vi "camera_synchrone_acquisition.vi"() -> ()   [LabVIEW 2018]
uses:
  <userlib>/WaveKit.lib/Controls/Image information.ctl
  <userlib>/WaveKit.lib/Controls/Image general information.ctl
  <userlib>/WaveKit.lib/Controls/Image acquisition information.ctl
  <userlib>/WaveKit.lib/Controls/Point2D.ctl
  <userlib>/WaveKit.lib/Controls/Data alignment enum.ctl
  <userlib>/WaveKit.lib/Classes/Camera/Camera.lvclass
  <userlib>/WaveKit.lib/Classes/CameraSet/CameraSet.lvclass
  <userlib>/WaveKit.lib/Classes/Image/Image.lvclass
panel:
  out "Acquisition information":T1={"Image general information"={"Camera serial number"="", "Smearing removed"=FALSE, "Background image removed"=FALSE, "Time Stamp"=timestamp(0 s since 1904-01-01), "Comment"="", "Camera_MAX_Level"=0}, "Acquisition information"={"Exposure duration (us)"=0, "Exposure duration specified (us)"=0, "Gain"=0.0, "Number of summed images"=0, "Trigger type"=""}, "Number of pixels"={"X"=0, "Y"=0}, "Number of bits"=enum."16"}
  in  "Init":bool
  in  "Reset error":bool
  in  "acquisition_mode":enum16{"last_image", "new_image"}(ring)
  out "exposure_duration_us (get)":u32
  in  "exposure_duration_us (set)":u32=1000 min=1
  out "Current error":errorcluster
  out "nb_image (get)":u32=10
  in  "nb_image (set)":u32=1 min=1
  in  "Show camera signal":bool
  in  "Exit":bool
  in  "Stop Acq":bool
  in  "Start Acq":bool
  out "Image Camera":u32[][](graph)
  in  "Configuration file path":path
  # "Acquisition Parameters"
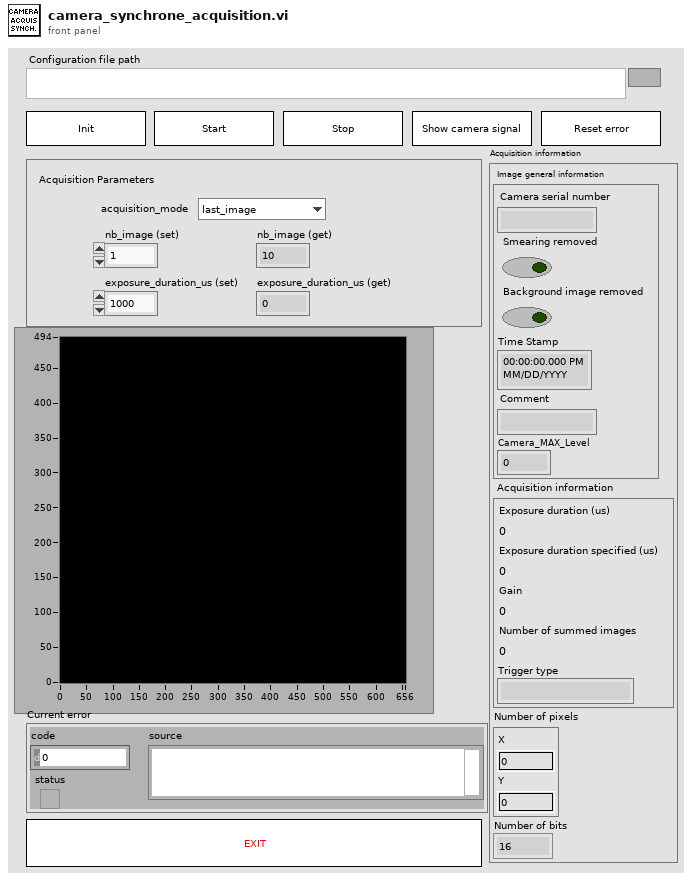
[diagram p1: front panel]
types:
  T1 = typedef "Image information.ctl" = cluster{"Image general information":T2, "Acquisition information":T3, "Number of pixels":T4, "Number of bits":T5}
  T2 = typedef "Image general information.ctl" = cluster{"Camera serial number":string, "Smearing removed":bool, "Background image removed":bool, "Time Stamp":timestamp, "Comment":string, "Camera_MAX_Level":i32}
  T3 = typedef "Image acquisition information.ctl" = cluster{"Exposure duration (us)":i32, "Exposure duration specified (us)":i32, "Gain":sgl, "Number of summed images":i32, "Trigger type":string}
  T4 = typedef "Point2D.ctl" = cluster{"X":u32, "Y":u32}
  T5 = typedef "Data alignment enum.ctl" = enum16{"8", "16", "32"}
  T6 = typedef "CameraSpecifications.ctl" = cluster{"Grabber name":string, "Camera name":string, "Camera sn":string, "Pixels_um":T7, "Maximum level":u32, "Data alignment":T5, "Is signed":bool, "Acquisition start":T4, "Acquisition length":T4, "MaxFrameRate_Hz":sgl, "Chip type":enum16{"Progressive scan", "Frame transfert"}}
  T7 = typedef "General dimensions definition.ctl" = cluster{"Size":T4, "Step":T8}
  T8 = typedef "Point2Df.ctl" = cluster{"X":sgl, "Y":sgl}
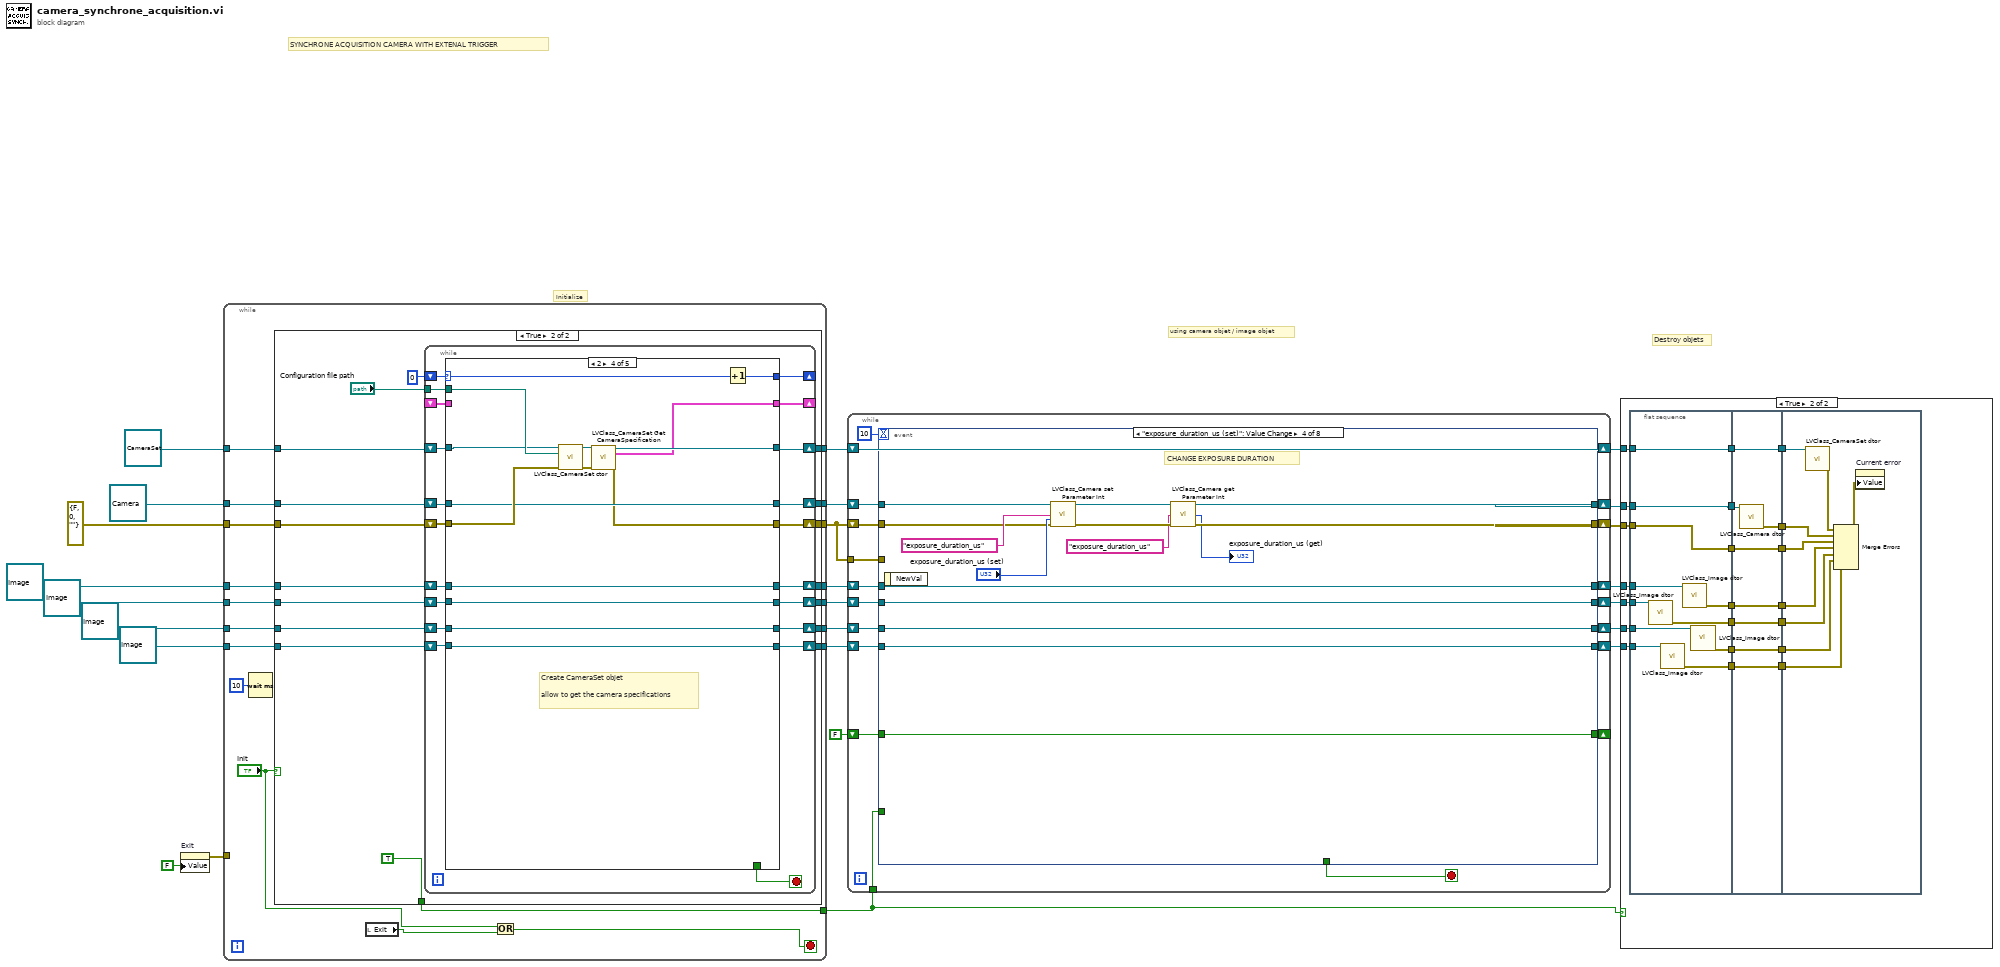
[diagram p0: block diagram]
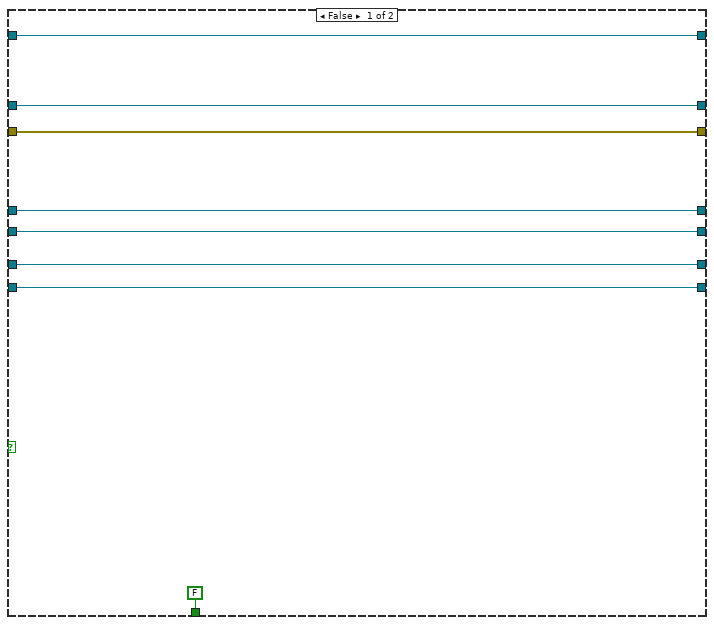
[diagram p3: hidden frame]
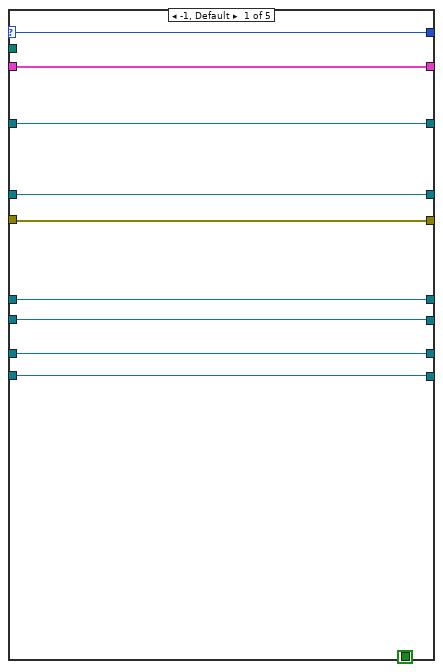
[diagram p4: hidden frame]
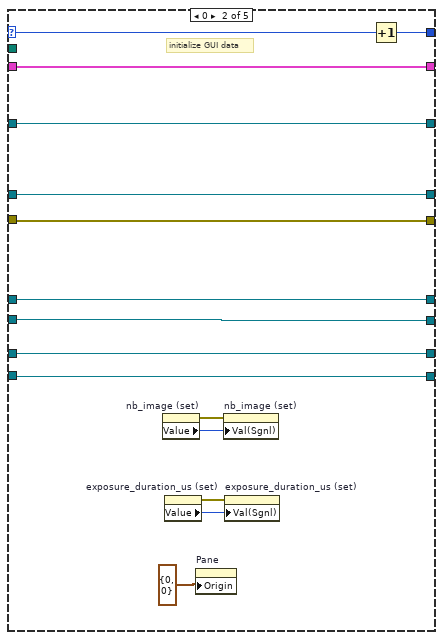
[diagram p5: hidden frame]
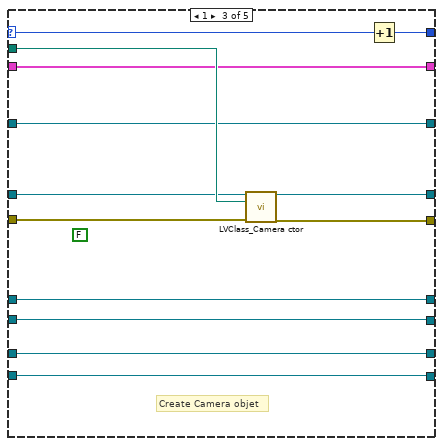
[diagram p6: hidden frame]
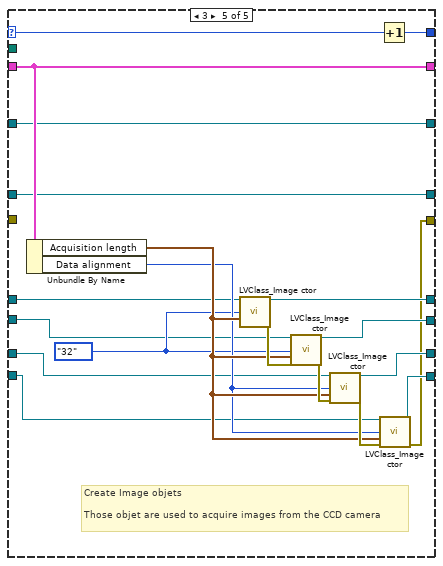
[diagram p7: hidden frame]
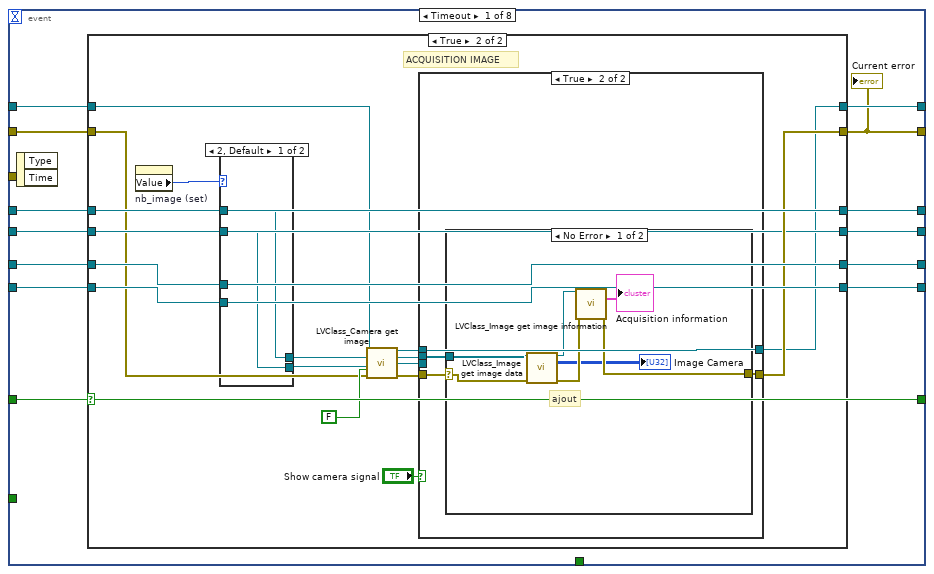
[diagram p8: hidden frame]
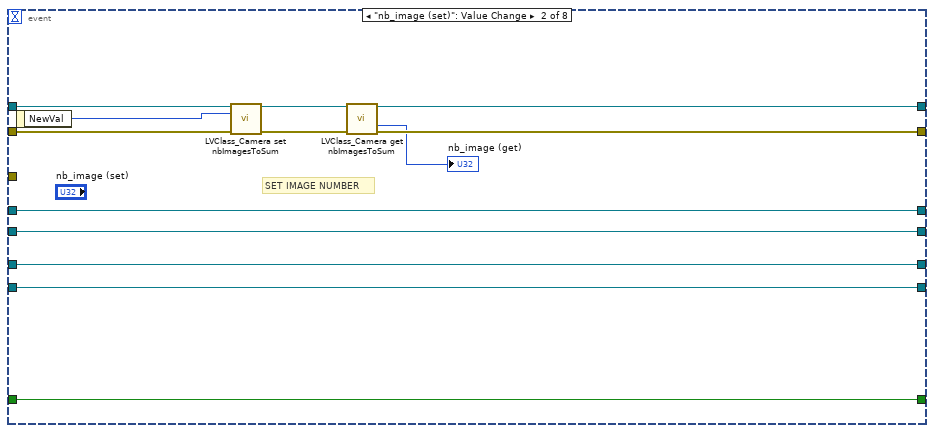
[diagram p13: hidden frame]
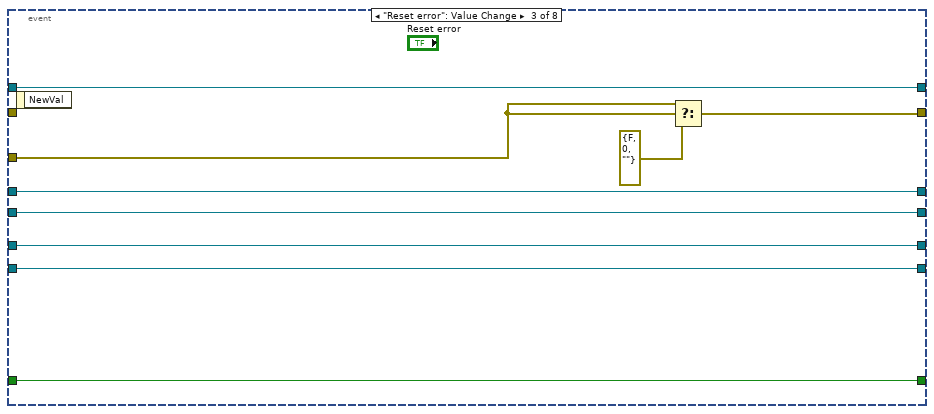
[diagram p14: hidden frame]
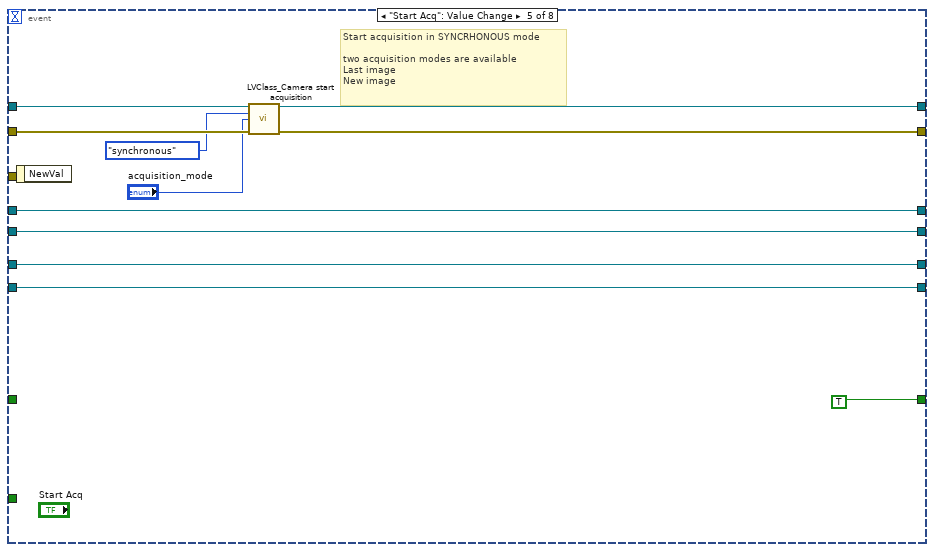
[diagram p15: hidden frame]
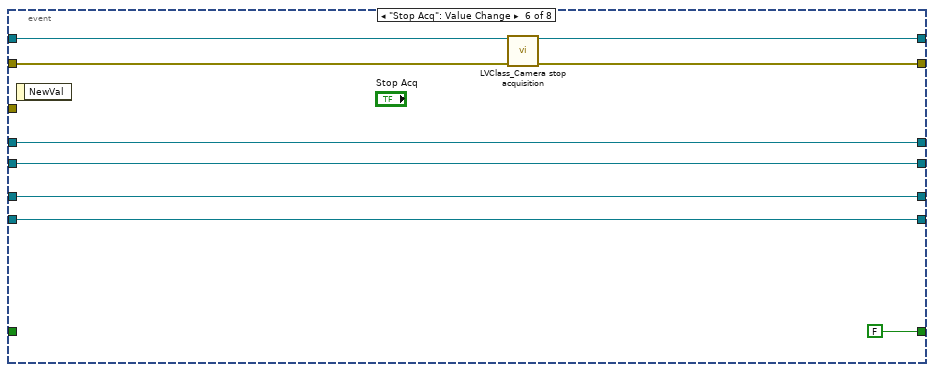
[diagram p16: hidden frame]
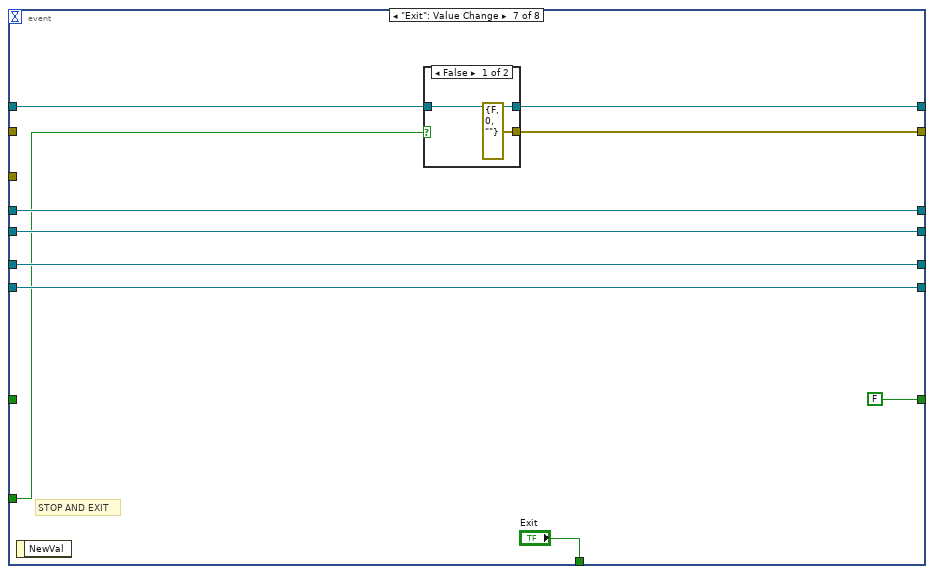
[diagram p17: hidden frame]
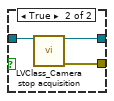
[diagram p18: hidden frame]
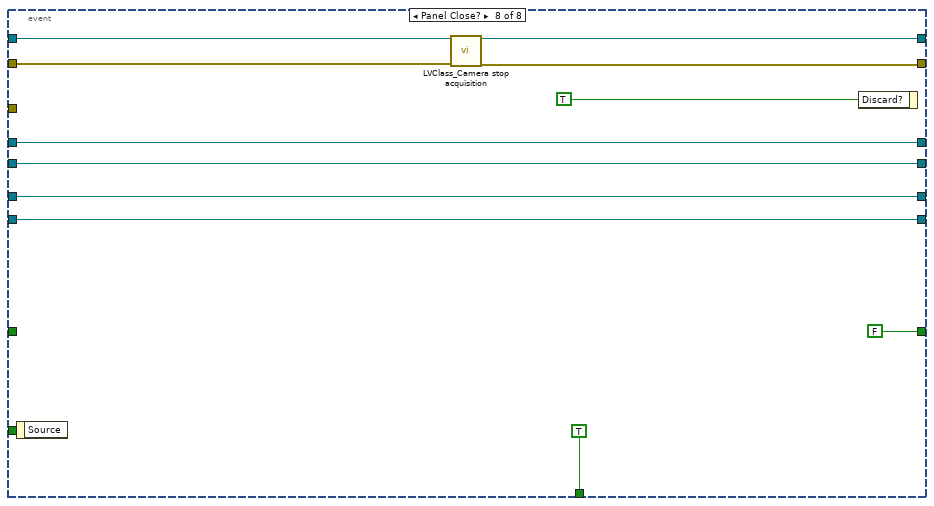
[diagram p19: hidden frame]
diagram:
  # "Destroy objets"
  # "using camera objet / image objet"
  # "Initialize"
  # "SYNCHRONE ACQUISITION CAMERA WITH EXTENAL TRIGGER"
  n1 = property on="Exit" class="Bool (strict)"("Value"=FALSE ("Exit")) -> (error out=w1:errorcluster)  [unwired: 2 in, 1 out]
  n2 = while {
    tunnel: [w44] -> w17
    tunnel: [w43] -> w16
    tunnel: [w42] -> w15
    tunnel: [w41] -> w14
    tunnel: [w40] -> w13
    tunnel: [w39] -> w12
    tunnel: refnum<class "Camera.lvclass"> refnum ("Camera.lvclass") -> [w38]
    tunnel: refnum<class "CameraSet.lvclass"> refnum ("CameraSet.lvclass") -> [w37]
    tunnel: refnum<class "Image.lvclass"> refnum ("Image in") -> [w36]
    tunnel: refnum<class "Image.lvclass"> refnum ("Image in") -> [w35]
    tunnel: refnum<class "Image.lvclass"> refnum ("Image in") -> [w34]
    tunnel: refnum<class "Image.lvclass"> refnum ("Image in") -> [w33]
    tunnel: errorcluster {"status"=FALSE, "code"=0, "source"=""} ("error out") -> [w32]
    tunnel: [w31] -> w4
    tunnel: [w27] -> w3
    tunnel: w1 -> [_]
    stop <- w28 stop-if-true
    n3 = Wait (ms)(milliseconds to wait=u32 10) -> ()  [unwired: 1 out]
    n4 = case shown="True" "Init" {
      tunnel: [w50 w69] -> w44
      tunnel: [w51 w68] -> w43
      tunnel: [w48 w66] -> w42
      tunnel: [w47 w65] -> w41
      tunnel: [w46 w64] -> w40
      tunnel: [w45 w63] -> w39
      tunnel: w38 -> [w50 w62]
      tunnel: w37 -> [w51 w60]
      tunnel: w36 -> [w48 w59]
      tunnel: w35 -> [w47 w58]
      tunnel: w34 -> [w46 w57]
      tunnel: w33 -> [w45 w56]
      tunnel: w32 -> [w49 w55]
      tunnel: [w49 w54] -> w31
      tunnel: [FALSE TRUE] -> w27
      frame False {
      }
      frame True {
        n5 = while {
          tunnel: "Configuration file path" -> [w87]
          shift-right: [w89] -> w69
          shift-left: w62 -> [w81]
          shift-right: [w71] -> _
          shift-left: 0 -> [w70]
          shift-right: [w88] -> w68
          shift-left: w60 -> [w80]
          shift-right: [w79] -> _
          shift-left: _ -> [w77]
          shift-right: [w86] -> w66
          shift-left: w59 -> [w78]
          shift-right: [w85] -> w65
          shift-left: w58 -> [w76]
          shift-right: [w84] -> w64
          shift-left: w57 -> [w74]
          shift-right: [w83] -> w63
          shift-left: w56 -> [w75]
          shift-right: [w82] -> w54
          shift-left: w55 -> [w72]
          stop <- w73 stop-if-true
          n6 = case shown="2" w70 {
            tunnel: [w99 w101 w127 w135 w149] -> w89
            tunnel: w87 -> [_ _ w126 w139 _]
            tunnel: [w98 w105 w124 w140 w150] -> w88
            tunnel: [w91 w106 w118 w130 w156] -> w86
            tunnel: [w92 w107 w119 w131 w155] -> w85
            tunnel: [w93 w108 w120 w132 w154] -> w84
            tunnel: [w94 w109 w121 w133 w153] -> w83
            tunnel: [w95 w100 w123 w134 w152] -> w82
            selector: w70 -> [w90 w103 w116 w129 w144]
            tunnel: w81 -> [w99 w101 w125 w135 w149]
            tunnel: w80 -> [w98 w105 w124 w138 w150]
            tunnel: [w96 w102 w122 w137 w151] -> w79
            tunnel: w78 -> [w91 w106 w118 w130 w148]
            tunnel: w77 -> [w96 w102 w122 _ w151]
            tunnel: w76 -> [w92 w107 w119 w131 w147]
            tunnel: w75 -> [w94 w109 w121 w133 w146]
            tunnel: w74 -> [w93 w108 w120 w132 w145]
            tunnel: [TRUE _ _ _ _] -> w73
            tunnel: w72 -> [w95 w100 w115 w136 _]
            tunnel: [w90 w104 w117 w128 w143] -> w71
            frame -1, Default {
            }
            frame 0 {
              # "initialize GUI data"
              n7 = property on="nb_image (set)" class="DigNum (strict)"() -> (error out=w114:errorcluster, "Value"=w113:u32)  [unwired: 2 in, 1 out]
              n8 = property on="exposure_duration_us (set)" class="DigNum (strict)"() -> (error out=w110:errorcluster, "Value"=w112:u32)  [unwired: 2 in, 1 out]
              n9 = property on="Pane" class="Pane"("Origin"=cluster{"Horizontal":i16, "Vertical":i16} {"Horizontal"=0, "Vertical"=0} ("Front Panel Window:Origin")) -> ()  [unwired: 2 in, 2 out]
              n10 = property on="nb_image (set)" class="DigNum (strict)"(error in=w114, "Val(Sgnl)"=w113) -> ()  [unwired: 1 in, 2 out]
              n11 = property on="exposure_duration_us (set)" class="DigNum (strict)"(error in=w110, "Val(Sgnl)"=w112) -> ()  [unwired: 1 in, 2 out]
              n12 = Increment(x=w103) -> (x+1=w104:i32)
            }
            frame 1 {
              (unwired) FALSE ("Acq required")
              # "Create Camera objet"
              n13 = call <userlib>:"LVClass_Camera ctor.vi"("Camera"=w125, "Configuration file path"=w126, "error in (no error)"=w115) -> ("Camera (new)"=w127:refnum<class "Camera.lvclass">, "error out"=w123:errorcluster)  [unwired: 11 in]
              n14 = Increment(x=w116) -> (x+1=w117:i32)
            }
            frame 2 {
              # "Create CameraSet objet\n\nallow to get the camera specifications"
              n15 = call <userlib>:"LVClass_CameraSet ctor.vi"("CameraSet.lvclass"=w138, "Configuration file path"=w139, "error in (no error)"=w136) -> ("CameraSet.lvclass"=w142:refnum<class "CameraSet.lvclass">, "error out"=w141:errorcluster)  [unwired: 11 in]
              n16 = call <userlib>:"LVClass_CameraSet Get CameraSpecification.vi"("CameraSet.lvclass"=w142, "error in (no error)"=w141) -> ("CameraSet.lvclass"=w140:refnum<class "CameraSet.lvclass">, "Camera Config"=w137:T6, "error out"=w134:errorcluster)  [unwired: 11 in]
              n17 = Increment(x=w129) -> (x+1=w128:i32)
            }
            frame 3 {
              w157 = Data_alignment_enum."32" ("Data alignment")
              # "Create Image objets\n\nThose objet are used to acquire images from the CCD camera"
              n18 = Unbundle By Name(w151) -> ("Acquisition length"=w159:T4, "Data alignment"=w158:T5)
              n19 = call <userlib>:"LVClass_Image ctor.vi"("Image in"=w148, "Data alignment"=w157, "Size"=w159) -> ("Image out"=w156:refnum<class "Image.lvclass">, "error out"=w160:errorcluster)  [unwired: 11 in]
              n20 = call <userlib>:"LVClass_Image ctor.vi"("Image in"=w147, "Data alignment"=w157, "Size"=w159, "error in (no error)"=w160) -> ("Image out"=w155:refnum<class "Image.lvclass">, "error out"=w161:errorcluster)  [unwired: 10 in]
              n21 = call <userlib>:"LVClass_Image ctor.vi"("Image in"=w145, "Data alignment"=w158, "Size"=w159, "error in (no error)"=w161) -> ("Image out"=w154:refnum<class "Image.lvclass">, "error out"=w162:errorcluster)  [unwired: 10 in]
              n22 = Increment(x=w144) -> (x+1=w143:i32)
              n23 = call <userlib>:"LVClass_Image ctor.vi"("Image in"=w146, "Data alignment"=w158, "Size"=w159, "error in (no error)"=w162) -> ("Image out"=w153:refnum<class "Image.lvclass">, "error out"=w152:errorcluster)  [unwired: 10 in]
            }
          }
        }
      }
    }
    n24 = local read "Exit"() -> (w29:bool)
    n25 = Or(x="Init", y=w29) -> (x .or. y?=w28:bool)
  }
  n26 = while {
    shift-right: [w178] -> w25
    shift-left: w4 -> [w180]
    shift-right: [w176] -> w24
    shift-left: w17 -> [w177]
    shift-right: [w170] -> w23
    shift-left: w15 -> [w175]
    shift-right: [w169] -> w22
    shift-left: w14 -> [w174]
    shift-right: [w168] -> w21
    shift-left: w13 -> [w173]
    shift-right: [w167] -> w20
    shift-left: w12 -> [w172]
    shift-right: [w166] -> _
    shift-left: FALSE -> [w171]
    shift-right: [w165] -> w19
    shift-left: w16 -> [w165]
    tunnel: w4 -> [w164]
    tunnel: w3 -> [w163]
    stop <- w179 stop-if-true
    n27 = event shown="[3] \"exposure_duration_us (set)\": Value Change" {
      selector: _ -> [_ _ _ _ _ _ _ _]
      dyn-events: _ -> [_ _ _ _ _ _ _ _]
      timeout: 10 -> [_ _ _ _ _ _ _ _]
      tunnel: w180 -> [w186 w247 _ w270 w282 w284 _ w309]
      tunnel: [_ _ _ _ _ _ "Exit" TRUE ("Exit")] -> w179
      tunnel: [w182 w245 w250 w265 w280 w290 w300 w314] -> w178
      tunnel: w177 -> [w191 w246 w252 w269 w283 w291 w301 w316]
      tunnel: [w190 w244 w252 w266 w281 w292 w299 w315] -> w176
      tunnel: w175 -> [w194 w237 w254 w259 w276 w286 w295 w310]
      tunnel: w174 -> [w193 w238 w255 w260 w275 w287 w296 w311]
      tunnel: w173 -> [w192 w239 w256 w261 w274 w288 w297 w312]
      tunnel: w172 -> [w187 w240 w257 w262 w273 w289 w298 w313]
      tunnel: w171 -> [w183 w236 w253 w258 _ _ _ _]
      tunnel: [w189 w237 w254 w259 w276 w286 w295 w310] -> w170
      tunnel: [w188 w238 w255 w260 w275 w287 w296 w311] -> w169
      tunnel: [w185 w239 w256 w261 w274 w288 w297 w312] -> w168
      tunnel: [w184 w240 w257 w262 w273 w289 w298 w313] -> w167
      tunnel: [w183 w236 w253 w258 TRUE FALSE FALSE FALSE] -> w166
      tunnel: w164 -> [_ _ w249 _ _ _ _ _]
      tunnel: w163 -> [_ _ _ _ _ _ w293 _]
      event Timeout {
        n28 = event-data() -> ()  [unwired: 1 in, 2 out]
        n29 = case shown="True" w183 {
          tunnel: [w195 w207] -> w182
          tunnel: w194 -> [w200 w213]
          tunnel: [w200 w213] -> w189
          tunnel: [w196 w204] -> w188
          tunnel: w192 -> [w199 w212]
          tunnel: w187 -> [w198 w211]
          tunnel: [w199 w212] -> w185
          tunnel: [w198 w211] -> w184
          tunnel: w193 -> [w196 w204]
          tunnel: w191 -> [w197 w203]
          tunnel: [w197 w202] -> w190
          tunnel: w186 -> [w195 w201]
          frame False {
          }
          frame True {
            # "ACQUISITION IMAGE"
            n30 = property on="nb_image (set)" class="DigNum (strict)"() -> ("Value"=w214:u32)  [unwired: 2 in, 2 out]
            n31 = case shown="2, Default" w214 {
              tunnel: [w219 w221] -> w215
              tunnel: w204 -> [w218 _]
              tunnel: w213 -> [w219 _]
              tunnel: [w218 w220] -> w210
              tunnel: w212 -> [_ w221]
              tunnel: w211 -> [_ w220]
              frame 2, Default {
              }
              frame 1 {
              }
            }
            n32 = call <userlib>:"LVClass_Camera get image.vi"("Camera in"=w203, "Image"=w215, "Image RAW"=w210, "remove_background"=FALSE, "error in (no error)"=w201) -> ("Camera out"=w217:refnum<class "Camera.lvclass">, "Image (dup)"=w208:refnum<class "Image.lvclass">, "Image (dup) RAW"=w209:refnum<class "Image.lvclass">, "error out"=w205:errorcluster)  [unwired: 7 in]
            n33 = case shown="True" "Show camera signal" {
              tunnel: w217 -> [w223 w224]
              tunnel: w208 -> [_ w225]
              tunnel: w205 -> [w222 w227]
              tunnel: [w223 w224] -> w202
              tunnel: [w222 w226] -> w207
              tunnel: w209 -> [_ _]
              frame False {
              }
              frame True {
                n34 = case shown="No Error" w227 {
                  selector: w227 -> [w234 w235]
                  tunnel: [w231 w235] -> w226
                  tunnel: w225 -> [w230 _]
                  frame No Error {
                    # "ajout"
                    n35 = call <userlib>:"LVClass_Image get image data.vi"("Image in"=w230, "error in (no error)"=w234) -> ("Image out"=w233:refnum<class "Image.lvclass">, "Image data out"=→"Image Camera":u32[][], "error out"=w232:errorcluster)  [unwired: 11 in]
                    n36 = call <userlib>:"LVClass_Image get image information.vi"("Image in"=w233, "error in (no error)"=w232) -> ("Acquisition information"=→"Acquisition information":T1, "error out"=w231:errorcluster)  [unwired: 11 in, 1 out]
                  }
                  frame Error {
                  }
                }
              }
            }
          }
        }
        "Current error" <- w182
      }
      event "nb_image (set)": Value Change {
        # "SET IMAGE NUMBER"
        n37 = event-data() -> ("NewVal"=w248:u32)  [unwired: 1 in]
        n38 = call <userlib>:"LVClass_Camera set nbImagesToSum.vi"("Camera in"=w246, "nb_image"=w248, "error in (no error)"=w247) -> ("Camera out"=w243:refnum<class "Camera.lvclass">, "error out"=w242:errorcluster)  [unwired: 11 in]
        n39 = call <userlib>:"LVClass_Camera get nbImagesToSum.vi"("Camera in"=w243, "error in (no error)"=w242) -> ("Camera out"=w244:refnum<class "Camera.lvclass">, "nb_image"=→"nb_image (get)":u32, "error out"=w245:errorcluster)  [unwired: 11 in]
      }
      event "Reset error": Value Change {
        n40 = event-data() -> ()  [unwired: 1 in, 1 out]
        n41 = Select(t=w249, s=w249, f=errorcluster {"status"=FALSE, "code"=0, "source"=""} ("error out")) -> (s? t:f=w250:errorcluster)
      }
      event "exposure_duration_us (set)": Value Change {
        # "CHANGE EXPOSURE DURATION"
        n42 = event-data() -> ()  [unwired: 1 in, 1 out]
        n43 = call <userlib>:"LVClass_Camera set Parameter Int.vi"("Camera in"=w269, "parameter_name"="exposure_duration_us", "value"="exposure_duration_us (set)", "error in (no error)"=w270) -> ("Camera out"=w268:refnum<class "Camera.lvclass">, "error out"=w267:errorcluster)  [unwired: 10 in]
        n44 = call <userlib>:"LVClass_Camera get Parameter Int.vi"("Camera in"=w268, "parameter_name"="exposure_duration_us", "error in (no error)"=w267) -> ("Camera out"=w266:refnum<class "Camera.lvclass">, "value"=→"exposure_duration_us (get)":i32, "error out"=w265:errorcluster)  [unwired: 10 in]
      }
      event "Start Acq": Value Change {
        # "Start acquisition in SYNCRHONOUS mode\n\ntwo acquisition modes are available\nLast image\nNew image"
        n45 = event-data() -> ()  [unwired: 1 in, 1 out]
        n46 = call <userlib>:"LVClass_Camera start acquisition.vi"("Camera in"=w283, "synchronisation_mode"=enum16{"synchronous", "asynchronous"}."synchronous", "acquisition_mode"="acquisition_mode", "error in (no error)"=w282) -> ("Camera out"=w281:refnum<class "Camera.lvclass">, "error out"=w280:errorcluster)  [unwired: 10 in]
      }
      event "Stop Acq": Value Change {
        n47 = event-data() -> ()  [unwired: 1 in, 1 out]
        n48 = call <userlib>:"LVClass_Camera stop acquisition.vi"("Camera in"=w291, "error in (no error)"=w284) -> ("Camera out"=w292:refnum<class "Camera.lvclass">, "error out"=w290:errorcluster)  [unwired: 12 in]
      }
      event "Exit": Value Change {
        # "STOP AND EXIT"
        n49 = event-data() -> ()  [unwired: 1 in, 1 out]
        n50 = case shown="False" w293 {
          tunnel: w301 -> [w304 w307]
          tunnel: [errorcluster {"status"=FALSE, "code"=0, "source"=""} ("error out") w306] -> w300
          tunnel: [w304 w305] -> w299
          frame False {
          }
          frame True {
            n51 = call <userlib>:"LVClass_Camera stop acquisition.vi"("Camera in"=w307) -> ("Camera out"=w305:refnum<class "Camera.lvclass">, "error out"=w306:errorcluster)  [unwired: 13 in]
          }
        }
      }
      event Panel Close? {
        n52 = event-data() -> ()  [unwired: 1 in, 1 out]
        n53 = call <userlib>:"LVClass_Camera stop acquisition.vi"("Camera in"=w316, "error in (no error)"=w309) -> ("Camera out"=w315:refnum<class "Camera.lvclass">, "error out"=w314:errorcluster)  [unwired: 12 in]
        n54 = event-data("Discard?"=TRUE) -> ()  [unwired: 1 in, 1 out]
      }
    }
  }
  n55 = case shown="True" w3 {
    tunnel: w25 -> [_ w325]
    tunnel: w24 -> [_ w324]
    tunnel: w23 -> [_ w323]
    tunnel: w22 -> [_ w322]
    tunnel: w21 -> [_ w321]
    tunnel: w20 -> [_ w320]
    tunnel: w19 -> [_ w319]
    frame False {
    }
    frame True {
      n56 = flat-sequence {
        tunnel: w324 -> [w350]
        tunnel: w325 -> [w348]
        tunnel: [w350] -> w339
        tunnel: w319 -> [w349]
        tunnel: [w349] -> w338
        tunnel: [w348] -> w337
        tunnel: w323 -> [w347]
        tunnel: w322 -> [w346]
        tunnel: w321 -> [w345]
        tunnel: w320 -> [w344]
        tunnel: [w343] -> w336
        tunnel: [w342] -> w335
        tunnel: [w341] -> w334
        tunnel: [w340] -> w333
        tunnel: w339 -> [w358]
        tunnel: w338 -> [w357]
        tunnel: w337 -> [w355]
        tunnel: [w357] -> w332
        tunnel: [w356] -> w331
        tunnel: [w355] -> w330
        tunnel: w336 -> [w354]
        tunnel: [w354] -> w329
        tunnel: w335 -> [w353]
        tunnel: [w353] -> w328
        tunnel: w334 -> [w352]
        tunnel: [w352] -> w327
        tunnel: w333 -> [w351]
        tunnel: [w351] -> w326
        tunnel: w332 -> [w367]
        tunnel: w331 -> [w365]
        tunnel: w330 -> [w364]
        tunnel: w329 -> [w363]
        tunnel: w328 -> [w362]
        tunnel: w327 -> [w361]
        tunnel: w326 -> [w360]
        frame #0 {
          n57 = call <userlib>:"LVClass_Image dtor.vi"("Image in"=w346) -> ("error out"=w342:errorcluster)  [unwired: 13 in, 1 out]
          n58 = call <userlib>:"LVClass_Image dtor.vi"("Image in"=w344) -> ("error out"=w340:errorcluster)  [unwired: 13 in, 1 out]
          n59 = call <userlib>:"LVClass_Image dtor.vi"("Image in"=w347) -> ("error out"=w343:errorcluster)  [unwired: 13 in, 1 out]
          n60 = call <userlib>:"LVClass_Image dtor.vi"("Image in"=w345) -> ("error out"=w341:errorcluster)  [unwired: 13 in, 1 out]
        }
        frame #1 {
          n61 = call <userlib>:"LVClass_Camera dtor.vi"("Camera in"=w358) -> ("error out"=w356:errorcluster)  [unwired: 13 in, 1 out]
        }
        frame #2 {
          n62 = call <userlib>:"LVClass_CameraSet dtor.vi"("CameraSet.lvclass"=w367) -> ("error out"=w366:errorcluster)  [unwired: 13 in, 1 out]
          n63 = Merge Errors(w366, w365, w364, w363, w362, w361, w360) -> (w359:errorcluster)
          n64 = property on="Current error" class="Clust (strict)"("Value"=w359) -> ()  [unwired: 2 in, 2 out]
        }
      }
    }
  }
